vi "Stop (uSMC).vi"(8 "error in (no error)":errorcluster, 9 "Index":i32, 11 "Visa array in":refnum<visa-resource-name>[](array[refnum])) -> (0 "error out":errorcluster, 3 "Visa array out":refnum<visa-resource-name>[](array[refnum]))   [LabVIEW 2010, in "SignalWriterMH110203USBStepperMotor.lvclass"]
uses:
  SignalWriterMH110203USBStepperMotor.lvclass
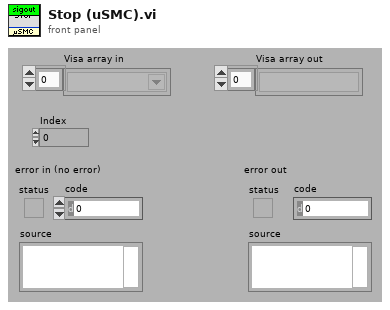
[diagram p1: front panel]
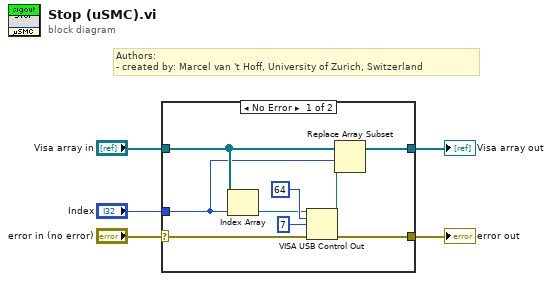
[diagram p0: block diagram]
diagram:
  # "Authors: \n- created by: Marcel van 't Hoff, University of Zurich, Switzerland"
  n1 = case shown="No Error" "error in (no error)" {
    selector: "error in (no error)" -> [w6 w16]
    tunnel: [w14 w16] -> w5
    tunnel: "Visa array in" -> [w10 w15]
    tunnel: "Index" -> [w9 _]
    tunnel: [w7 w15] -> w2
    frame No Error {
      n2 = Index Array(array=w10, index=w9) -> (element=w11:refnum<visa-resource-name>)
      n3 = VISA USB Control Out(0:w11, 5:i16 64 ("request type"), 7:i16 7 ("request type"), 11:w6) -> (4:w8:refnum<visa-resource-name>, 15:w14:errorcluster)  [unwired: 3 in]
      n4 = Replace Array Subset(array=w10, new element=w8, index=w9) -> (w7:refnum<visa-resource-name>[])
    }
    frame Error {
    }
  }
  "error out" <- w5
  "Visa array out" <- w2
